vi "AdventofCodeDay2.vi"() -> ()   [LabVIEW 2019]
panel:
  out "Solution 2":u32
  out "Solution 1":u32
  in  "String":string
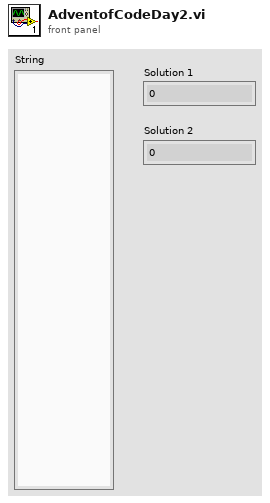
[diagram p1: front panel]
types:
  T1 = enum16{"Native", "Native Command Line", "UNIX", "Macintosh", "DOS"}
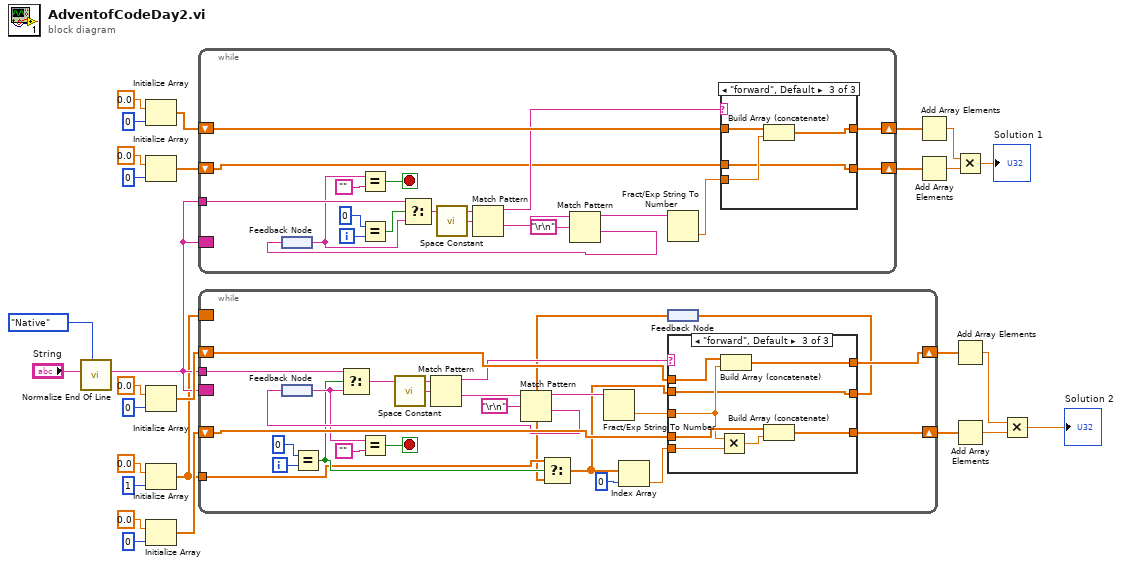
[diagram p0: block diagram]
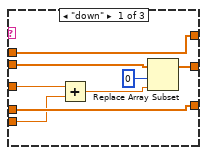
[diagram p2: hidden frame]
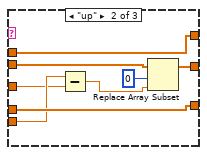
[diagram p3: hidden frame]
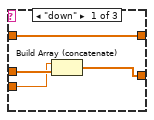
[diagram p4: hidden frame]
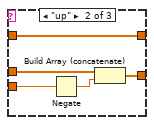
[diagram p5: hidden frame]
diagram:
  n1 = call <vilib>:"Normalize End Of Line.vi"("end of line (Native)"=T1."Native", "string in"="String") -> ("string out"=w4:string)  [unwired: 6 in]
  n2 = Initialize Array(0.0 ("element"), 0 ("dimension size")) -> (w24:dbl[])
  n3 = Initialize Array(0.0 ("element"), 0 ("dimension size")) -> (w21:dbl[])
  n4 = Initialize Array(0.0 ("element"), 0 ("dimension size")) -> (w6:dbl[])
  n5 = Initialize Array(0.0 ("element"), 1 ("dimension size")) -> (w1:dbl[])
  n6 = Initialize Array(0.0 ("element"), 0 ("dimension size")) -> (w5:dbl[])
  n7 = while {
    tunnel: w4 -> [w31]
    shift-right: [w42] -> w20
    shift-left: w24 -> [w43]
    shift-right: [w38] -> w19
    shift-left: w21 -> [w39]
    border: w4 -> [_]
    i -> [w35]
    stop <- w36 stop-if-true
    n8 = feedback #1() -> (w29:string)
    n9 = Equal?(x=w29, y="") -> (x = y?=w36:bool)
    n10 = Equal?(x=0, y=w35) -> (x = y?=w33:bool)
    n11 = Select(t=w31, s=w33, f=w29) -> (s? t:f=w32:string)
    n12 = call <vilib>:"Space Constant.vi"() -> ("String"=w41:string)
    n13 = Match Pattern(string=w32, regular expression=w41) -> (before substring=w40:string, after substring=w46:string)  [unwired: 1 in, 2 out]
    n14 = Match Pattern(string=w46, regular expression="\r\n") -> (before substring=w45:string, after substring=w30:string)  [unwired: 1 in, 2 out]
    n15 = feedback-in #1(w30) -> ()
    n16 = Fract/Exp String To Number(string=w45) -> (number=w44:dbl)  [unwired: 3 in, 1 out]
    n17 = case shown="\"forward\", Default" w40 {
      tunnel: w44 -> [w48 w53 w59]
      tunnel: w43 -> [w49 w56 w60]
      tunnel: [w49 w56 w58] -> w42
      tunnel: w39 -> [w51 w55 w57]
      tunnel: [w50 w54 w57] -> w38
      frame "down" {
        n18 = Build Array (concatenate)(w48, w51) -> (w50:dbl[])
      }
      frame "up" {
        n19 = Negate(x=w53) -> (-x=w52:dbl)
        n20 = Build Array (concatenate)(w55, w52) -> (w54:dbl[])
      }
      frame "forward", Default {
        n21 = Build Array (concatenate)(w60, w59) -> (w58:dbl[])
      }
    }
  }
  n22 = while {
    tunnel: w4 -> [w70]
    shift-right: [w80] -> w15
    shift-left: w6 -> [w81]
    border: w4 -> [_]
    tunnel: w1 -> [w66]
    border: w1 -> [_]
    shift-right: [w76] -> w14
    shift-left: w5 -> [w77]
    i -> [w73]
    stop <- w74 stop-if-true
    n23 = feedback #2() -> (w68:string)
    n24 = Equal?(x=0, y=w73) -> (x = y?=w67:bool)
    n25 = Select(t=w70, s=w67, f=w68) -> (s? t:f=w71:string)
    n26 = Equal?(x=w68, y="") -> (x = y?=w74:bool)
    n27 = call <vilib>:"Space Constant.vi"() -> ("String"=w79:string)
    n28 = Match Pattern(string=w71, regular expression=w79) -> (before substring=w78:string, after substring=w84:string)  [unwired: 1 in, 2 out]
    n29 = Match Pattern(string=w84, regular expression="\r\n") -> (before substring=w83:string, after substring=w69:string)  [unwired: 1 in, 2 out]
    n30 = feedback-in #2(w69) -> ()
    n31 = Fract/Exp String To Number(string=w83) -> (number=w82:dbl)  [unwired: 3 in, 1 out]
    n32 = feedback #3() -> (w65:dbl[])
    n33 = Select(t=w66, s=w67, f=w65) -> (s? t:f=w62:dbl[])
    n34 = Index Array(array=w62, index=0) -> (element=w64:dbl)
    n35 = case shown="\"forward\", Default" w78 {
      tunnel: w82 -> [w92 w94 w106]
      tunnel: w81 -> [w93 w101 w109]
      tunnel: [w93 w101 w108] -> w80
      tunnel: w77 -> [w91 w99 w107]
      tunnel: [w91 w99 w104] -> w76
      tunnel: w64 -> [w90 w95 w103]
      tunnel: w62 -> [w89 w97 w102]
      tunnel: [w86 w96 w102] -> w61
      frame "down" {
        n36 = Add(x=w92, y=w90) -> (x+y=w88:dbl)
        n37 = Replace Array Subset(array=w89, new element=w88, index=0) -> (w86:dbl[])
      }
      frame "up" {
        n38 = Subtract(x=w95, y=w94) -> (x-y=w98:dbl)
        n39 = Replace Array Subset(array=w97, new element=w98, index=0) -> (w96:dbl[])
      }
      frame "forward", Default {
        n40 = Multiply(x=w106, y=w103) -> (x*y=w105:dbl)
        n41 = Build Array (concatenate)(w109, w106) -> (w108:dbl[])
        n42 = Build Array (concatenate)(w107, w105) -> (w104:dbl[])
      }
    }
    n43 = feedback-in #3(w61) -> ()
  }
  n44 = Add Array Elements(numeric array=w20) -> (sum=w17:dbl)
  n45 = Add Array Elements(numeric array=w19) -> (sum=w18:dbl)
  n46 = Multiply(x=w17, y=w18) -> (x*y=→"Solution 1":dbl)
  n47 = Add Array Elements(numeric array=w15) -> (sum=w12:dbl)
  n48 = Add Array Elements(numeric array=w14) -> (sum=w13:dbl)
  n49 = Multiply(x=w12, y=w13) -> (x*y=→"Solution 2":dbl)
